vi "AutoFocus.vi"(2 "error in (no error)":errorcluster, 3 "path":path=path "C:/Users/light/Desktop/ReadParam") -> (0 "error out":errorcluster)   [LabVIEW 2014]
uses:
  <vilib>/Utility/config.llb/Write Key (I32).vi
  <vilib>/Utility/config.llb/Read Key (I32).vi
  <vilib>/Utility/config.llb/NI_LVConfig.lvlib
panel:
  # "1: end"
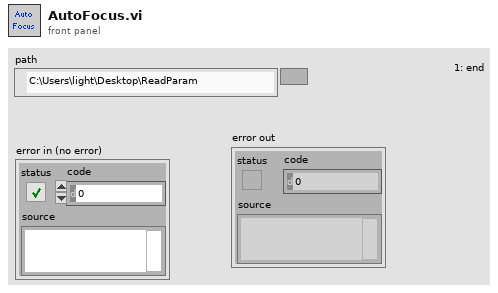
[diagram p1: front panel]
types:
  T1 = typedef "NI_LVConfig.lvlib/Config Data RefNum.ctl" = refnum<k1>
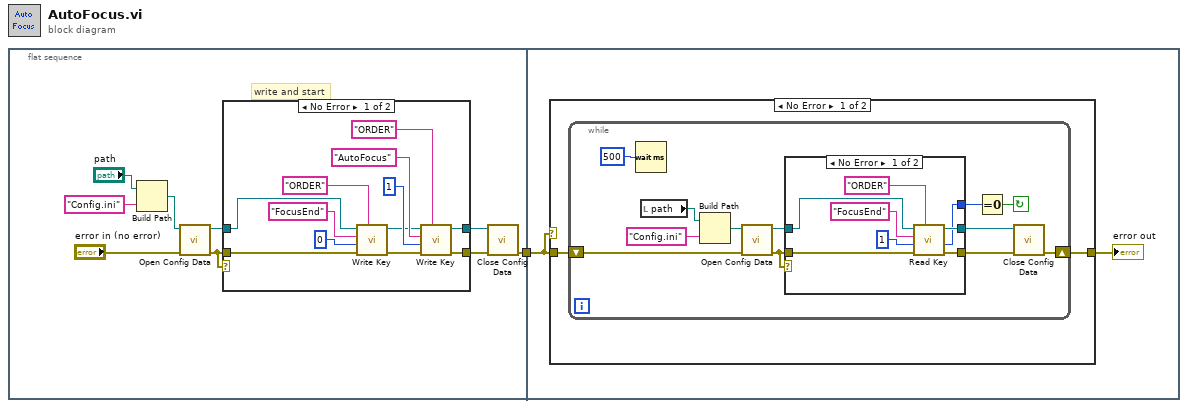
[diagram p0: block diagram]
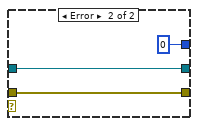
[diagram p3: hidden frame]
diagram:
  n1 = flat-sequence {
    tunnel: [w2] -> w1
    tunnel: w1 -> [w26]
    frame #0 {
      # "write and start"
      n2 = Build Path(base path="path", name or relative path="Config.ini") -> (appended path=w4:path)
      n3 = call <vilib>:"Open Config Data.vi"("error in (no error)"="error in (no error)", "configuration file path"=w4) -> ("error out"=w8:errorcluster, "refnum"=w7:T1)  [unwired: 7 in, 1 out]
      n4 = case shown="No Error" w8 {
        tunnel: [w12 w23] -> w10
        tunnel: [w11 w24] -> w9
        tunnel: w8 -> [w14 w24]
        tunnel: w7 -> [w13 w23]
        frame No Error {
          n5 = call-poly <vilib>:"Write Key.vi"("section"="ORDER", "error in (no error)"=w14, "value"=0 ("default value"), "key"="FocusEnd", "refnum"=w13) -> ("error out"=w15:errorcluster, "refnum out"=w16:T1)  [unwired: 4 in, 1 out]
          n6 = call-poly <vilib>:"Write Key.vi"("section"="ORDER", "error in (no error)"=w15, "value"=1 ("default value"), "key"="AutoFocus", "refnum"=w16) -> ("error out"=w11:errorcluster, "refnum out"=w12:T1)  [unwired: 4 in, 1 out]
        }
        frame Error {
        }
      }
      n7 = call <vilib>:"Close Config Data.vi"("error in (no error)"=w9, "refnum"=w10) -> ("error out"=w2:errorcluster)  [unwired: 8 in, 1 out]
    }
    frame #1 {
      n8 = case shown="No Error" w26 {
        tunnel: w26 -> [w28 w52]
        tunnel: [w27 w52] -> w25
        frame No Error {
          n9 = while {
            shift-right: [w29] -> w27
            shift-left: w28 -> [w30]
            stop <- w32 continue-if-true
            n10 = Wait (ms)(milliseconds to wait=u32 500) -> ()  [unwired: 1 out]
            n11 = local read "path"() -> (w35:path)
            n12 = Build Path(base path=w35, name or relative path="Config.ini") -> (appended path=w36:path)
            n13 = call <vilib>:"Open Config Data.vi"("error in (no error)"=w30, "configuration file path"=w36) -> ("error out"=w39:errorcluster, "refnum"=w40:T1)  [unwired: 7 in, 1 out]
            n14 = case shown="No Error" w39 {
              tunnel: [w43 w51] -> w38
              tunnel: w39 -> [w46 w51]
              tunnel: w40 -> [w45 w50]
              tunnel: [w42 w50] -> w34
              tunnel: [w41 0 ("value")] -> w33
              frame No Error {
                n15 = call-poly <vilib>:"Read Key.vi"("section"="ORDER", "error in (no error)"=w46, "default value"=1, "key"="FocusEnd", "refnum"=w45) -> ("error out"=w43:errorcluster, "value"=w41:i32, "refnum out"=w42:T1)  [unwired: 3 in, 1 out]
              }
              frame Error {
              }
            }
            n16 = Equal To 0?(x=w33) -> (x = 0?=w32:bool)
            n17 = call <vilib>:"Close Config Data.vi"("error in (no error)"=w38, "refnum"=w34) -> ("error out"=w29:errorcluster)  [unwired: 8 in, 1 out]
          }
        }
        frame Error {
        }
      }
      "error out" <- w25
    }
  }
